vi "Test_API_AddSink_NoError.vi"(8 "error in (no error)":errorcluster, 11 "TestCase in":refnum<class "TestLocalLogInstance.lvclass">) -> (0 "error out":errorcluster, 3 "TestCase out":refnum<class "TestLocalLogInstance.lvclass">)   [LabVIEW 2017, in "TestLocalLogInstance.lvclass"]
uses:
  TestLocalLogInstance.lvclass
  Source/Composed Log/LoggerReference/LoggerReference.lvclass/LoggerReference.ctl
  9d660762-14d6-4a5f-8cc2-8fea042b4442.vi
  ce3293c4-4e8f-466b-b20c-c1ab2ef8c7cf.vi
  Source/Composed Log/LoggerReference/Return Aggregate Queues.vi
  Source/Composed Log/LoggerReference/Add Aggregate Log.vi
  9d660762-14d6-4a5f-8cc2-8fea042b4442.vi/b3726afd-6f82-43ec-95a2-0632910b4503.vi
  Source/Composed Log/LoggerReference/Send Add Sink.vi
  Source/LVQueue Sink/LVQueue Sink.lvclass
  C:/CS/Internal/LabVIEW/Logger/Source/Composed Log/Log Sink/Log Sink.lvclass
  Source/Composed Log/Application Logger/Launch Worker Loop.vi
  Source/Composed Log/LoggerReference/Initialize Logger Instance.vi
  Source/Composed Log/LoggerReference/LoggerReference.lvclass
  Source/Composed Log/IErrorFormat/IErrorFormat.lvclass
  Source/Composed Log/Log Sink/Log Sink.lvclass
  <vilib>/addons/_JKI Toolkits/VI Tester/TestCase.llb/TestCase.lvclass
  C:/Program Files (x86)/National Instruments/LabVIEW 2017/vi.lib/addons/_JKI Toolkits/VI Tester/TestCase.llb/TestCase.lvclass
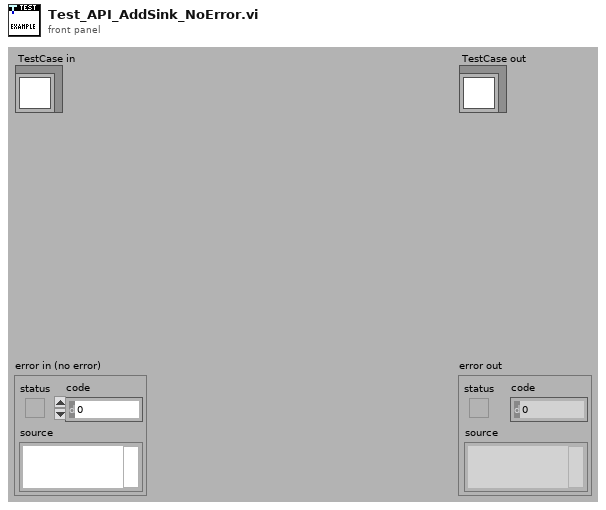
[diagram p1: front panel]
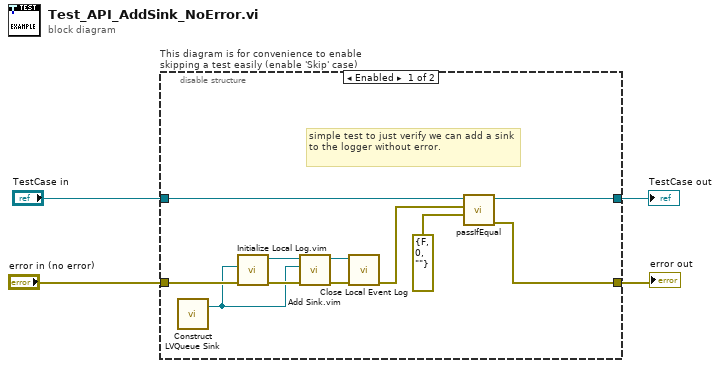
[diagram p0: block diagram]
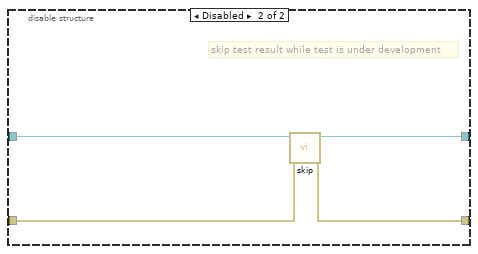
[diagram p2: hidden frame]
diagram:
  n1 = disable-structure "This diagram is for convenience to enable skipping a test easily (enable 'Skip' case)" shown="Enabled" {
    disable-tunnel: "TestCase in" -> [w14 w19]
    disable-tunnel: [w15 w17] -> w1
    disable-tunnel: [w12 w18] -> w3
    disable-tunnel: "error in (no error)" -> [w11 w16]
    frame Enabled {
      # "simple test to just verify we can add a sink to the logger without error."
      n2 = call "Construct LVQueue Sink.vi"() -> ("LVQueue Sink out"=w5:refnum<class "LVQueue Sink.lvclass">)  [unwired: 10 in, 1 out]
      n3 = call "Initialize Local Log.vim"("error in (no error)"=w11, "Startup Sink(s)"=w5) -> ("error out"=w10:errorcluster, "Log Instance Reference"=w9:refnum<class "LoggerReference.lvclass">)  [unwired: 7 in, 1 out]
      n4 = call "Add Sink.vim"("error in (no error)"=w10, "Log Sink(s)"=w5, "Log Instance In"=w9) -> ("error out"=w7:errorcluster, "Log Instance Out"=w8:refnum<class "LoggerReference.lvclass">)  [unwired: 6 in, 1 out]
      n5 = call "Close Local Event Log.vi"("error in (no error)"=w7, "Log Instance"=w8) -> ("error out"=w6:errorcluster)  [unwired: 9 in]
      n6 = call-dynamic "passIfEqual.vi"("y"=errorcluster {"status"=FALSE, "code"=0, "source"=""} ("error out"), "x"=w6, "TestCase in"=w14) -> ("error out"=w12:errorcluster, "TestCase out"=w15:refnum<class "TestLocalLogInstance.lvclass">)  [unwired: 7 in]
    }
    frame Disabled {
      # "skip test result while test is under development"
      n7 = call <vilib>:"skip.vi"("error in (no error)"=w16, "TestCase in"=w19) -> ("error out"=w18:errorcluster, "TestCase out"=w17:refnum<class "TestLocalLogInstance.lvclass">)  [unwired: 8 in]
    }
  }
  "error out" <- w3
  "TestCase out" <- w1
